vi "StringToAutoData.vi"(11 "String":string) -> (3 "Auto":T1)   [LabVIEW 2017]
uses:
  AutoFileDataType.ctl
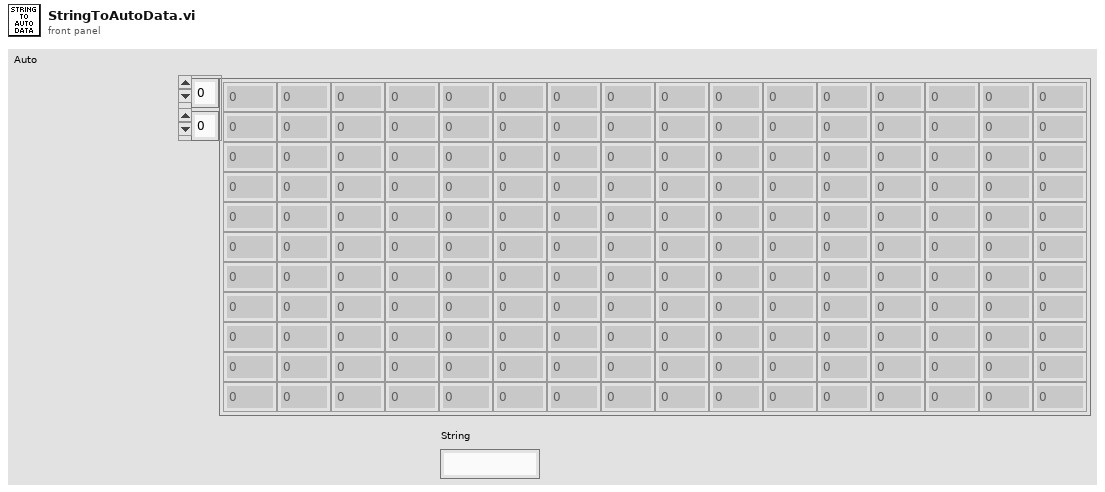
[diagram p1: front panel]
types:
  T1 = typedef "AutoFileDataType.ctl" = dbl[][]
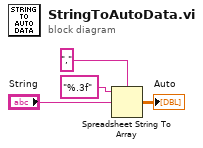
[diagram p0: block diagram]
diagram:
  n1 = Spreadsheet String To Array(delimiter (Tab)=",", format string="%.3f", spreadsheet string="String") -> (array=→"Auto":dbl[][])  [unwired: 1 in]
